vi "坐标平移.vi"() -> ()   [LabVIEW 2018]
uses:
  <vilib>/Analysis/coordinate.llb/2D Cartesian Coordinate Shift (Array).vi
  <vilib>/Analysis/NI_AALPro.lvlib
panel:
  in  "停止":bool
  out "Y2":dbl[](graph)
  out "X2":dbl[](graph)
  out "Y":dbl[](graph)
  out "X":dbl[](graph)
  in  "shift":cluster{"dx":dbl, "dy":dbl} caption="位移"
  in  "Y":dbl[](array[numeric])
  in  "X":dbl[](array[numeric])
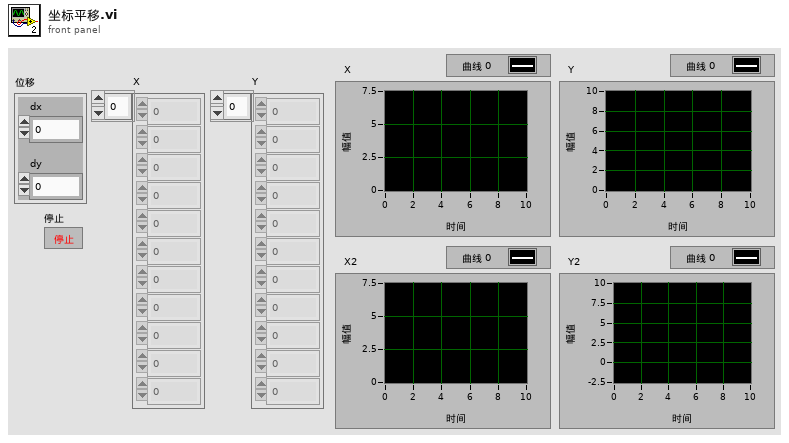
[diagram p1: front panel]
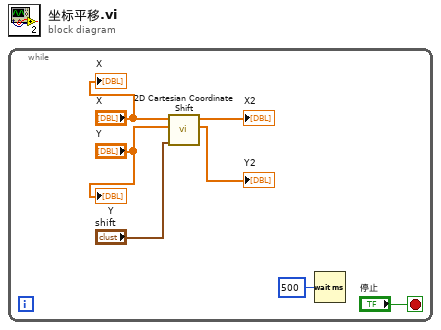
[diagram p0: block diagram]
diagram:
  n1 = while {
    stop <- "停止" stop-if-true
    n2 = call-poly <vilib>:"2D Cartesian Coordinate Shift.vi"("shift"="shift", "Y"="Y", "X"="X") -> ("Y Out"=→"Y2":dbl[], "X Out"=→"X2":dbl[])  [unwired: 6 in, 1 out]
    n3 = Wait (ms)(milliseconds to wait=u32 500 ("等待时间（毫秒）")) -> ()  [unwired: 1 out]
    "X" <- "X"
    "Y" <- "Y"
  }
